vi "Set Voltage Level.vi"(6 "low level":dbl, 8 "error in (no error)":errorcluster, 9 "level (V)":dbl, 10 "channel list":string, 11 "instrument handle":refnum<k15>) -> (0 "error out":errorcluster, 3 "instrument handle out":refnum<k15>)   [LabVIEW 2018]
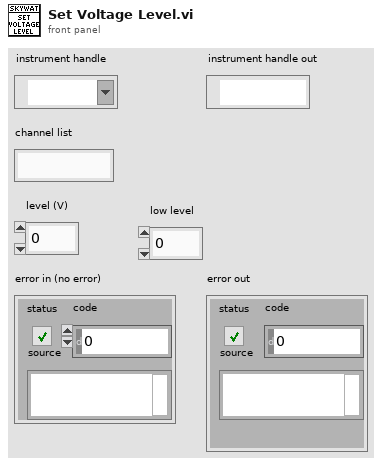
[diagram p1: front panel]
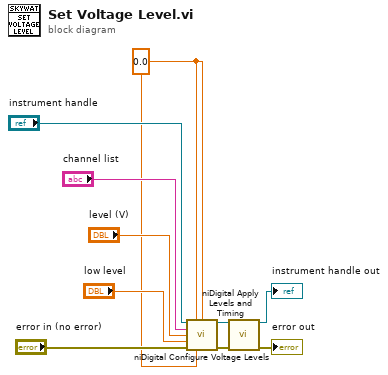
[diagram p0: block diagram]
diagram:
  w1 = 0.0 ("vterm (V)")
  n1 = call <instrlib>:"niDigital Configure Voltage Levels.vi"("instrument handle"="instrument handle", "vol (V)"=w1, "voh (V)"=w1, "channel list"="channel list", "vih (V)"="level (V)", "vil (V)"="low level", "error in"="error in (no error)", "vterm (V)"=w1) -> ("instrument handle out"=w6:refnum<k15>, "error out"=w5:errorcluster)  [unwired: 6 in]
  n2 = call <instrlib>:"niDigital Apply Levels and Timing.vi"("instrument handle"=w6, "error in"=w5) -> ("instrument handle out"=→"instrument handle out":refnum<k15>, "error out"=→"error out":errorcluster)  [unwired: 12 in]
